vi "PSK_Mod_Transmit_test_Q_ulyd_funker.vi"() -> ()   [LabVIEW 2014]
uses:
  <vilib>/addons/Modulation/Analog/controls/Complex Data Waveform.ctl
  <vilib>/addons/Modulation/Digital/General/MT Generate Bits (Galois, PN Order).vi
  <vilib>/addons/Modulation/Digital/Support/Common/Validators/mod_Generate Bits Validate.vi
  <vilib>/addons/Modulation/Analog/support/mod_Set Error Source.vi
  <vilib>/addons/Modulation/Digital/General/MT Generate PSK System Parameters(M).vi
  <vilib>/addons/Modulation/Digital/Support/Common/Validators/mod_Generate Filter Coefficients Validate.vi
  <vilib>/addons/Modulation/Digital/General/subVIs/mod_Generate Filter Coefficients.vi
  <vilib>/addons/Modulation/Digital/General/subVIs/mod_Generate Bits PN Sequence.vi
  <vilib>/addons/Modulation/Digital/General/MT Generate Bits (User Defined).vi
  <instrlib>/niUSRP/niUSRP Write Tx Data (CDB Cluster).vi
  <vilib>/addons/Modulation/niDMT.lvlib
  <vilib>/addons/Modulation/niAMT.lvlib
panel:
  in  "stop":bool
  in  "Packet Parameters":T1={"Length of sync sequence (20)"=20, "Number of message bits"=128, "Number of guardbits"=40, "PN sequence order (31)"=31, "Number of packets in burst"=40}
  out "Before demod&compensation":waveform(dbl)(graph)
  out "Constellation Graph":T2(graph) caption="Tx Signal Constellation"
  out "bits sent":i32
  out "input bit stream":i8[](array[numeric]) caption="input package"
  out "time/packet":dbl
  out "output bit stream":i8[](array[numeric])
  in  "error in (no error)":errorcluster
  out "error out":errorcluster
  in  "USRP IP address":refnum<k15>="192.168.10.1"
  in  "Tx Parameters":T3={"Tx IQ Sampling\nRate [s/sec]"=400000.0, "Tx Frequency [Hz]"=5795000000.0, "Tx Gain [dB]"=0.0, "Tx Antenna"="TX1"} {"Tx Gain [dB]" format="%#.6p"; "Tx Frequency [Hz]" format="%#.6p"; "Tx IQ Sampling\nRate [s/sec]" format="%#.6p"}
  out "Actual Tx Parameters":T3={"Tx IQ Sampling\nRate [s/sec]"=400000.0, "Tx Frequency [Hz]"=915000000.0, "Tx Gain [dB]"=0.0, "Tx Antenna"="TX1"} {"Tx Gain [dB]" format="%#.6p"; "Tx Frequency [Hz]" format="%#.6p"; "Tx IQ Sampling\nRate [s/sec]" format="%#.6p"}
  in  "filter parameters":T4={"Alpha"=0.5, "Filter Length"=6, "TX Filter"=enum."Root Raised Cos"} {"Alpha" format="%.2f"}
  in  "QPSK System Parameters":T5={"Samples per Symbol"=8, "symbol map"=[], "Differential PSK"=enum."disable", "PSK type"=0} {"PSK type" items=["normal", "shifted", "offset"]; "symbol map" format="%.3f"}
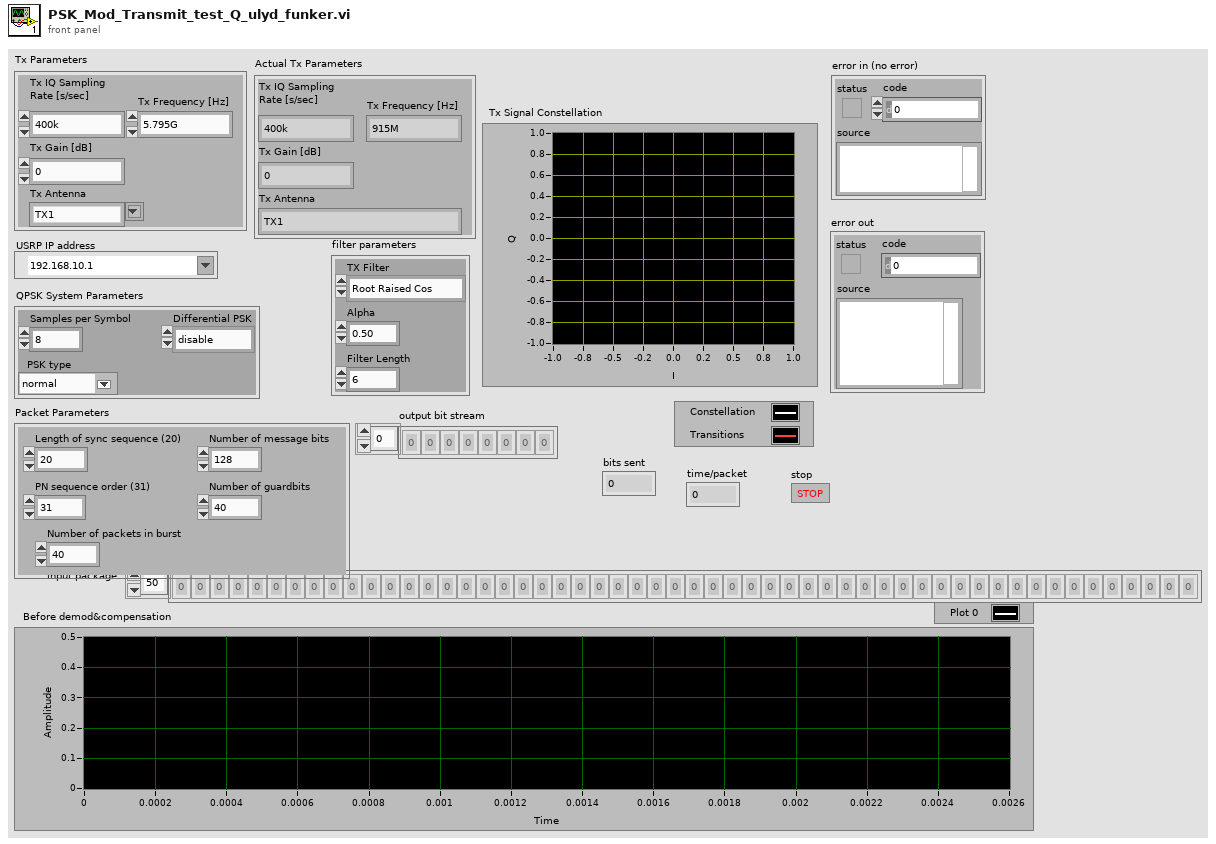
[diagram p1: front panel]
types:
  T1 = cluster{"Length of sync sequence (20)":i32, "Number of message bits":i32, "Number of guardbits":i32, "PN sequence order (31)":i32, "Number of packets in burst":i32}
  T2 = cluster{"constellation":dbl[], "oversampled data":dbl[]}[]
  T3 = cluster{"Tx IQ Sampling\nRate [s/sec]":dbl, "Tx Frequency [Hz]":dbl, "Tx Gain [dB]":dbl, "Tx Antenna":string}
  T4 = cluster{"Alpha":dbl, "Filter Length":i32, "TX Filter":enum16{"none", "Raised Cosine", "Root Raised Cos", "Gaussian"}}
  T5 = cluster{"Samples per Symbol":i32, "symbol map":cdb[], "Differential PSK":enum16{"disable", "enable"}, "PSK type":u16}
  T6 = typedef "niAMT.lvlib/Complex Data Waveform.ctl" = cluster{"t0":dbl, "dt":dbl, "Y":cdb[]}
  T7 = enum16{"FSK", "PSK", "QAM", "MSK", "PAM", "ASK", "CPM"}
  T8 = enum16{"none", "Raised Cosine", "Root Raised Cos", "Gaussian"}
  T9 = cluster{"samples per symbol (16)":i32, "symbol map":cdb[], "differential PSK":enum16{"disable", "enable"}, "PSK type":u16}
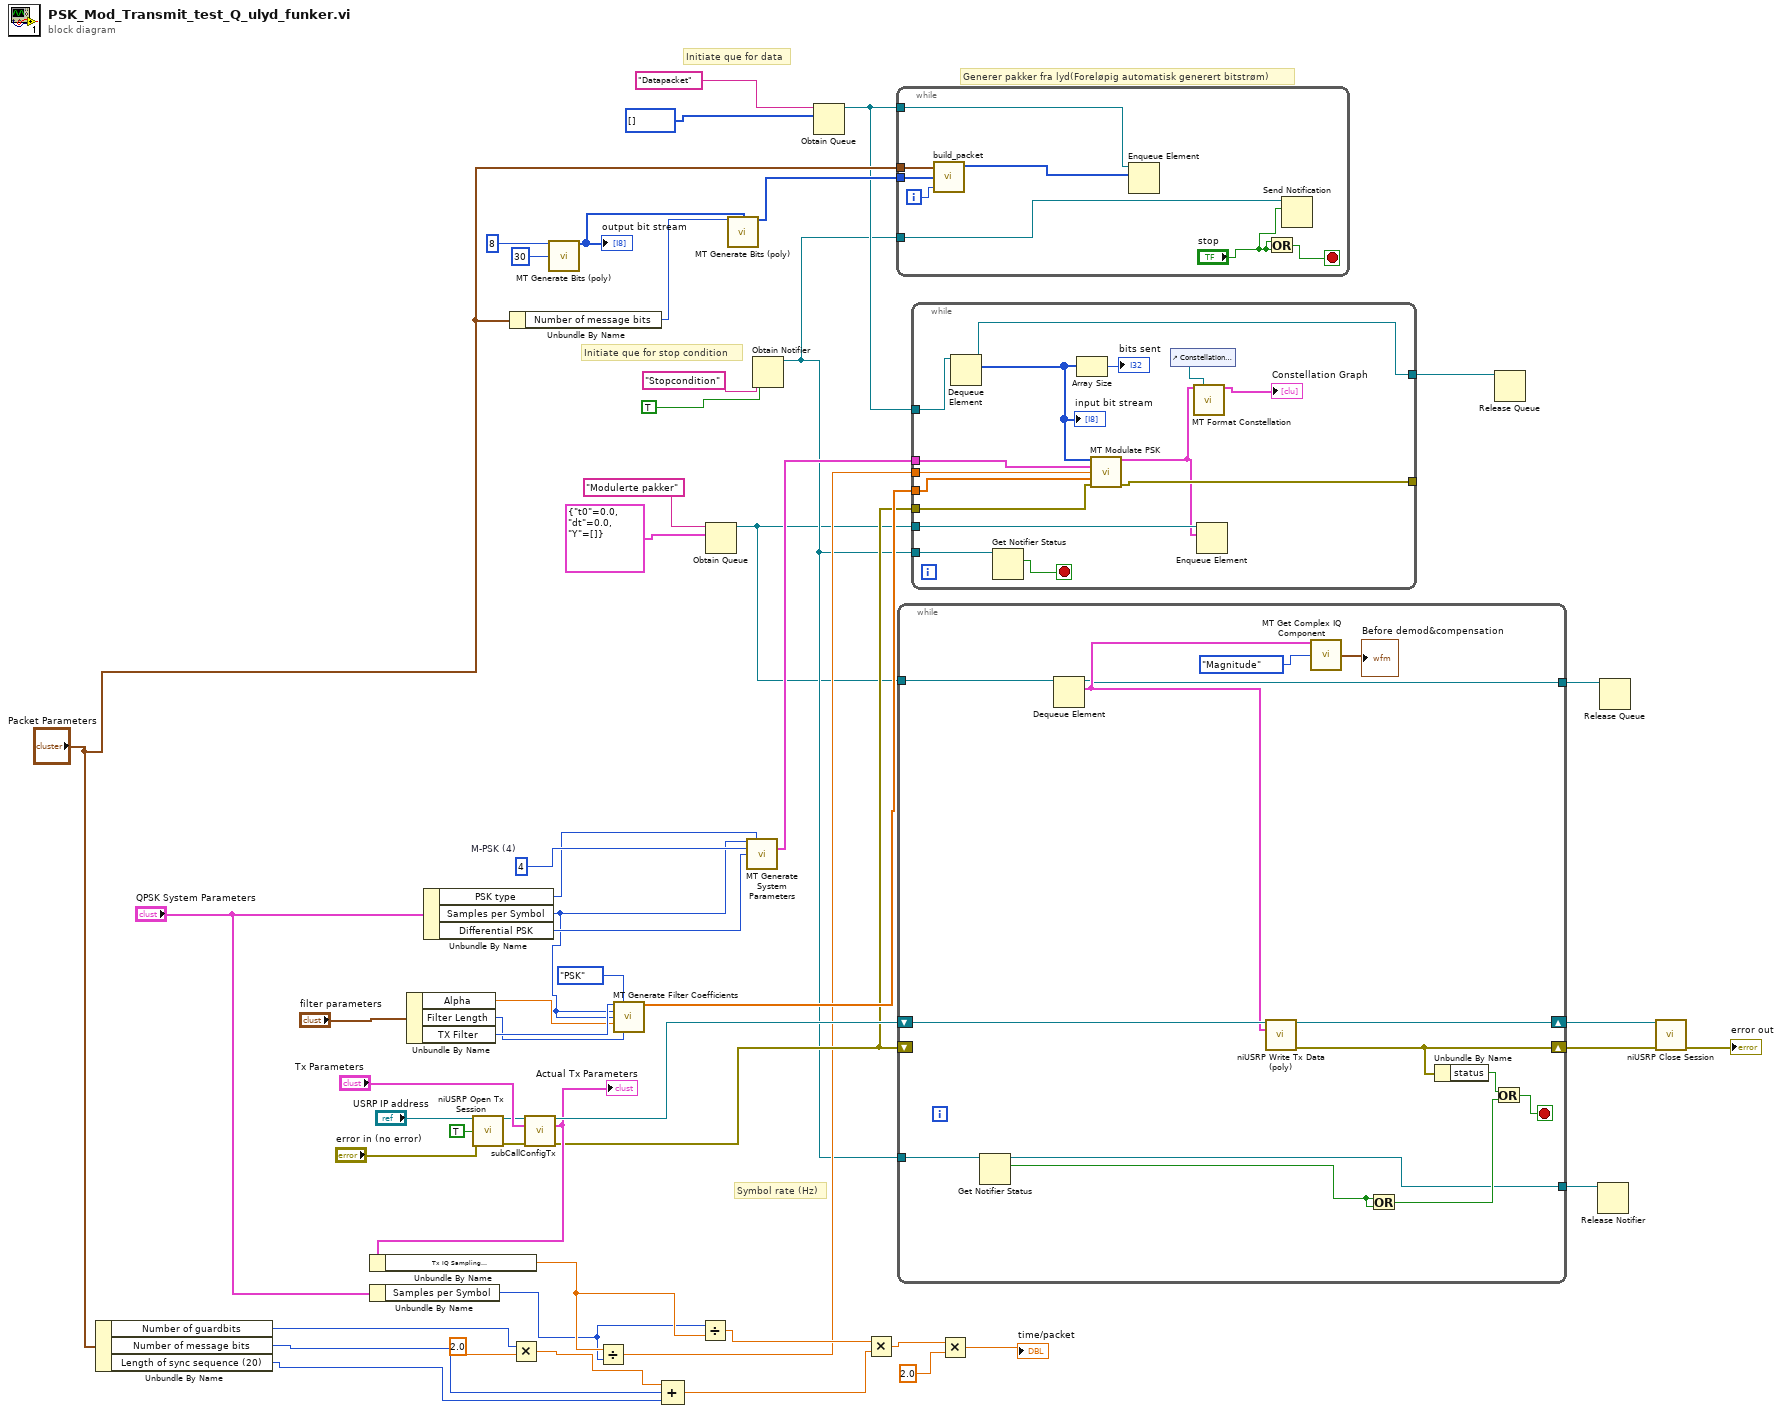
[diagram p0: block diagram]
diagram:
  w54 = 4  # M-PSK (4)
  # "Initiate que for stop condition"
  # "Initiate que for data"
  # "Generer pakker fra lyd(Foreløpig automatisk generert bitstrøm)"
  # "Symbol rate (Hz)"
  n1 = Unbundle By Name("Packet Parameters") -> ("Number of guardbits"=w25:i32, "Number of message bits"=w15:i32, "Length of sync sequence (20)"=w23:i32)
  n2 = Unbundle By Name("QPSK System Parameters") -> ("Samples per Symbol"=w22:i32)
  n3 = Unbundle By Name("filter parameters") -> ("Alpha"=w50:dbl, "Filter Length"=w51:i32, "TX Filter"=w52:T8)
  n4 = Unbundle By Name("QPSK System Parameters") -> ("PSK type"=w53:u16, "Samples per Symbol"=w32:i32, "Differential PSK"=w55:enum16{"disable", "enable"})
  n5 = call <instrlib>:"niUSRP Open Tx Session.vi"("device names"="USRP IP address", "reset"=TRUE, "error in (no error)"="error in (no error)") -> ("session handle out"=w46:refnum<k15>, "error out"=w45:errorcluster)  [unwired: 11 in]
  n6 = Unbundle By Name("Packet Parameters") -> ("Number of message bits"=w18:i32)
  n7 = Multiply(x=w25, y=2.0 ("x")) -> (x*y=w33:dbl)
  n8 = call "subCallConfigTx.vi"("session handle"=w46, "Tx Parameters"="Tx Parameters", "error in"=w45) -> ("session handle out"=w40:refnum<k15>, "Actual Tx Parameters"=w37:T3, "error out"=w8:errorcluster)  [unwired: 10 in]
  "Actual Tx Parameters" <- w37
  n9 = Unbundle By Name(w37) -> ("Tx IQ Sampling\nRate [s/sec]"=w31:dbl)
  n10 = call-poly <vilib>:"MT Generate Bits (poly).vi"("total bits (128)"=8, "PN sequence order (9)"=30) -> ("output bit stream"=w36:i8[])  [unwired: 11 in, 2 out]
  "output bit stream" <- w36
  n11 = Divide(x=w31, y=w22) -> (x/y=w6:dbl)
  n12 = call <vilib>:"MT Generate Filter Coefficients.vi"("pulse shaping filter (none)"=w52, "modulation type"=T7."PSK", "pulse shaping samples per symbol (16)"=w32, "matched samples per symbol (16)"=w32, "filter parameter"=w50, "filter length (symbols)"=w51) -> ("pulse shaping filter coefficients"=w9:dbl[])  [unwired: 7 in, 2 out]
  n13 = Compound Arithmetic op=ADD(w33, w15, w23) -> (w29:dbl)
  n14 = Divide(x=w22, y=w31) -> (x/y=w30:dbl)
  n15 = Obtain Queue(name (unnamed)="Modulerte pakker", element data type=T6 {"t0"=0.0, "dt"=0.0, "Y"=[]} ("output complex waveform")) -> (queue out=w2:refnum<queue>)  [unwired: 3 in, 2 out]
  n16 = call-poly <vilib>:"MT Generate Bits (poly).vi"("total bits (128)"=w18, "user base bit pattern"=w36) -> ("output bit stream"=w16:i8[])  [unwired: 12 in, 1 out]
  n17 = call-poly <vilib>:"MT Generate System Parameters.vi"("samples per symbol (16)"=w32, "PSK type"=w53, "M-PSK (4)"=w54, "differential PSK"=w55) -> ("PSK system parameters"=w7:T9)  [unwired: 9 in, 2 out]
  n18 = Obtain Notifier(name (unnamed)="Stopcondition", notification data type=TRUE ("stop 2")) -> (notifier out=w5:refnum<notifier>)  [unwired: 2 in, 2 out]
  n19 = Obtain Queue(name (unnamed)="Datapacket", element data type=i8[] [] ("output bitstream")) -> (queue out=w11:refnum<queue>)  [unwired: 3 in, 2 out]
  n20 = Multiply(x=w30, y=w29) -> (x*y=w27:dbl)
  n21 = while {
    tunnel: "Packet Parameters" -> [w63]
    tunnel: w16 -> [w61]
    tunnel: w11 -> [w60]
    tunnel: w5 -> [w57]
    i -> [w62]
    stop <- w58 stop-if-true
    n22 = call "build_packet.vi"("Packet number"=w62, "message data"=w61, "Packet Parameters"=w63) -> ("output bitstream"=w59:i8[])  [unwired: 5 in]
    n23 = Enqueue Element(queue=w60, element=w59) -> ()  [unwired: 2 in, 3 out]
    n24 = Or(x="stop", y="stop") -> (x .or. y?=w58:bool)
    n25 = Send Notification(notification="stop", notifier=w57) -> ()  [unwired: 1 in, 2 out]
  }
  n26 = while {
    shift-right: [w72] -> w38
    shift-left: w8 -> [_]
    shift-right: [w73] -> w39
    shift-left: w40 -> [w71]
    tunnel: w5 -> [w68]
    tunnel: [w67] -> w12
    tunnel: w2 -> [w66]
    tunnel: [w64] -> w1
    stop <- w76 stop-if-true
    n27 = Get Notifier Status(notifier=w68) -> (notifier out=w67:refnum<notifier>, current notification=w69:bool)  [unwired: 1 in, 3 out]
    n28 = Dequeue Element(queue=w66) -> (queue out=w64:refnum<queue>, element=w65:T6)  [unwired: 2 in, 2 out]
    n29 = call-poly <instrlib>:"niUSRP Write Tx Data (poly).vi"("session handle"=w71, "data"=w65) -> ("session handle out"=w73:refnum<k15>, "error out"=w72:errorcluster)  [unwired: 12 in]
    n30 = call <vilib>:"MT Get Complex IQ Component.vi"("IQ data (complex) in"=w65, "component choice"=enum16{"I", "Q", "Magnitude", "Phase"}."Magnitude") -> ("CE component"=→"Before demod&compensation":waveform(dbl))  [unwired: 11 in, 2 out]
    n31 = Or(x=w69, y=w69) -> (x .or. y?=w70:bool)
    n32 = Unbundle By Name(w72) -> ("status"=w77:bool)
    n33 = Or(x=w77, y=w70) -> (x .or. y?=w76:bool)
  }
  n34 = while {
    tunnel: w11 -> [w92]
    tunnel: [w91] -> w10
    tunnel: w9 -> [w87]
    tunnel: w8 -> [w86]
    tunnel: [w85] -> _
    tunnel: w7 -> [w84]
    tunnel: w6 -> [w83]
    tunnel: w5 -> [w81]
    tunnel: w2 -> [w79]
    stop <- w80 stop-if-true
    n35 = Dequeue Element(queue=w92) -> (queue out=w91:refnum<queue>, element=w82:i8[])  [unwired: 2 in, 2 out]
    "input bit stream" <- w82
    n36 = Get Notifier Status(notifier=w81) -> (current notification=w80:bool)  [unwired: 1 in, 4 out]
    n37 = Array Size(array=w82) -> (size(s)=→"bits sent":i32)
    n38 = call <vilib>:"MT Modulate PSK.vi"("input bit stream"=w82, "PSK system parameters"=w84, "symbol rate (Hz)"=w83, "pulse shaping filter coefficients"=w87, "error in (no error)"=w86) -> ("output complex waveform"=w78:T6, "error out"=w85:errorcluster)  [unwired: 8 in, 1 out]
    n39 = control-ref of="Constellation Graph"() -> (w88:refnum<vi>)
    n40 = call <vilib>:"MT Format Constellation.vi"("waveform"=w78, "constellation reference"=w88) -> ("constellation graph"=→"Constellation Graph":T2)  [unwired: 12 in, 1 out]
    n41 = Enqueue Element(queue=w79, element=w78) -> ()  [unwired: 2 in, 3 out]
  }
  n42 = Multiply(x=w27, y=2.0) -> (x*y=→"time/packet":dbl)
  n43 = Release Queue(queue=w10) -> ()  [unwired: 2 in, 3 out]
  n44 = Release Notifier(notifier=w12) -> ()  [unwired: 2 in, 3 out]
  n45 = Release Queue(queue=w1) -> ()  [unwired: 2 in, 3 out]
  n46 = call <instrlib>:"niUSRP Close Session.vi"("session handle"=w39, "error in (no error)"=w38) -> ("error out"=→"error out":errorcluster)  [unwired: 13 in]
